vi "conversor-hex-car.vi"(10 "String":string) -> (2 "String 2":string)   [LabVIEW 2019]
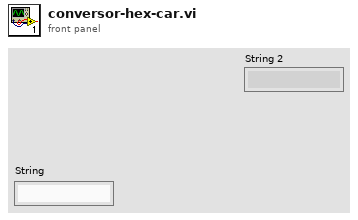
[diagram p1: front panel]
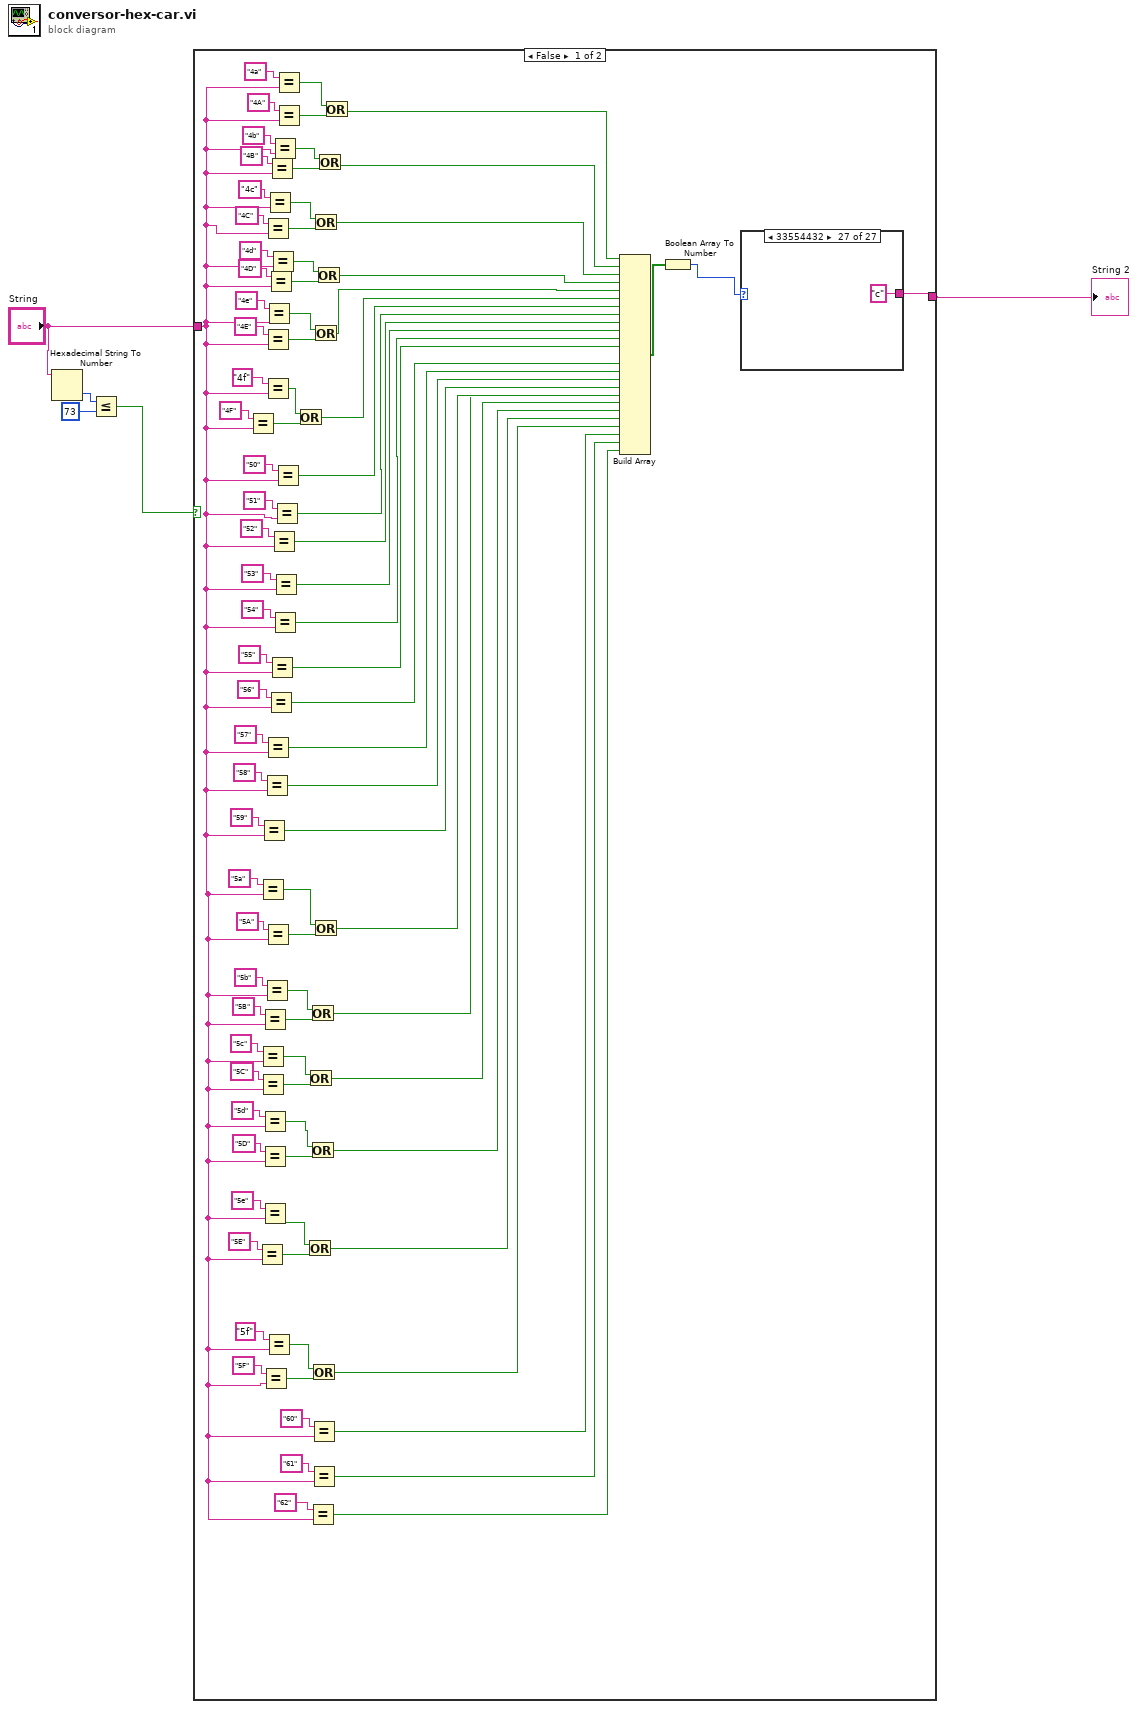
[diagram p0: block diagram]
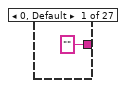
[diagram p2: hidden frame]
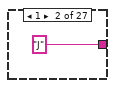
[diagram p3: hidden frame]
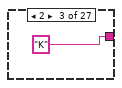
[diagram p4: hidden frame]
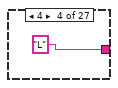
[diagram p5: hidden frame]
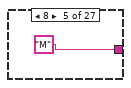
[diagram p6: hidden frame]
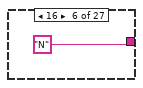
[diagram p7: hidden frame]
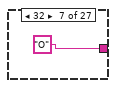
[diagram p8: hidden frame]
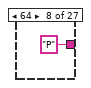
[diagram p9: hidden frame]
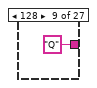
[diagram p10: hidden frame]
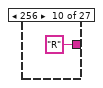
[diagram p11: hidden frame]
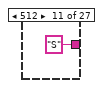
[diagram p12: hidden frame]
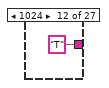
[diagram p13: hidden frame]
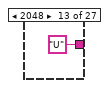
[diagram p14: hidden frame]
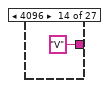
[diagram p15: hidden frame]
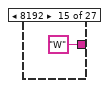
[diagram p16: hidden frame]
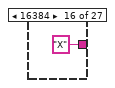
[diagram p17: hidden frame]
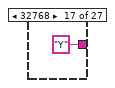
[diagram p18: hidden frame]
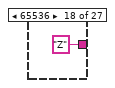
[diagram p19: hidden frame]
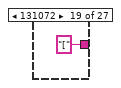
[diagram p20: hidden frame]
diagram:
  n1 = Hexadecimal String To Number(string="String") -> (number=w5:u32)  [unwired: 2 in, 1 out]
  n2 = Less Or Equal?(x=w5, y=u32 73) -> (x <= y?=w3:bool)
  n3 = case shown="False" w3 {
    tunnel: [w56 w188] -> w1
    tunnel: "String" -> [w8 w125]
    frame False {
      n4 = Equal?(x="4F", y=w8) -> (x = y?=w34:bool)
      n5 = Equal?(x="5E", y=w8) -> (x = y?=w14:bool)
      n6 = Equal?(x="5a", y=w8) -> (x = y?=w28:bool)
      n7 = Equal?(x="5c", y=w8) -> (x = y?=w20:bool)
      n8 = Equal?(x="5C", y=w8) -> (x = y?=w22:bool)
      n9 = Equal?(x="59", y=w8) -> (x = y?=w69:bool)
      n10 = Equal?(x="5B", y=w8) -> (x = y?=w26:bool)
      n11 = Equal?(x="5d", y=w8) -> (x = y?=w16:bool)
      n12 = Equal?(x="5D", y=w8) -> (x = y?=w18:bool)
      n13 = Equal?(x="5e", y=w8) -> (x = y?=w12:bool)
      n14 = Equal?(x="5F", y=w8) -> (x = y?=w10:bool)
      n15 = Equal?(x="58", y=w8) -> (x = y?=w70:bool)
      n16 = Equal?(x="5b", y=w8) -> (x = y?=w24:bool)
      n17 = Equal?(x="4C", y=w8) -> (x = y?=w46:bool)
      n18 = Equal?(x="4E", y=w8) -> (x = y?=w38:bool)
      n19 = Equal?(x="4f", y=w8) -> (x = y?=w32:bool)
      n20 = Equal?(x="57", y=w8) -> (x = y?=w71:bool)
      n21 = Equal?(x="5A", y=w8) -> (x = y?=w30:bool)
      n22 = Equal?(x="4e", y=w8) -> (x = y?=w36:bool)
      n23 = Equal?(x="5f", y=w8) -> (x = y?=w7:bool)
      n24 = Equal?(x="4c", y=w8) -> (x = y?=w44:bool)
      n25 = Equal?(x="4D", y=w8) -> (x = y?=w42:bool)
      n26 = Equal?(x="56", y=w8) -> (x = y?=w72:bool)
      n27 = Equal?(x="4B", y=w8) -> (x = y?=w50:bool)
      n28 = Equal?(x="55", y=w8) -> (x = y?=w77:bool)
      n29 = Equal?(x="4d", y=w8) -> (x = y?=w40:bool)
      n30 = Equal?(x="52", y=w8) -> (x = y?=w80:bool)
      n31 = Equal?(x="4b", y=w8) -> (x = y?=w48:bool)
      n32 = Equal?(x="54", y=w8) -> (x = y?=w78:bool)
      n33 = Equal?(x="53", y=w8) -> (x = y?=w79:bool)
      n34 = Equal?(x="51", y=w8) -> (x = y?=w81:bool)
      n35 = Equal?(x="50", y=w8) -> (x = y?=w82:bool)
      n36 = Equal?(x="4a", y=w8) -> (x = y?=w52:bool)
      n37 = Equal?(x="4A", y=w8) -> (x = y?=w54:bool)
      n38 = Or(x=w32, y=w34) -> (x .or. y?=w31:bool)
      n39 = Or(x=w12, y=w14) -> (x .or. y?=w11:bool)
      n40 = Or(x=w20, y=w22) -> (x .or. y?=w19:bool)
      n41 = Or(x=w24, y=w26) -> (x .or. y?=w23:bool)
      n42 = Or(x=w16, y=w18) -> (x .or. y?=w15:bool)
      n43 = Equal?(x="62", y=w8) -> (x = y?=w57:bool)
      n44 = Or(x=w7, y=w10) -> (x .or. y?=w6:bool)
      n45 = Equal?(x="60", y=w8) -> (x = y?=w59:bool)
      n46 = Equal?(x="61", y=w8) -> (x = y?=w58:bool)
      n47 = Or(x=w44, y=w46) -> (x .or. y?=w43:bool)
      n48 = Or(x=w36, y=w38) -> (x .or. y?=w35:bool)
      n49 = Or(x=w28, y=w30) -> (x .or. y?=w27:bool)
      n50 = Or(x=w40, y=w42) -> (x .or. y?=w39:bool)
      n51 = Or(x=w48, y=w50) -> (x .or. y?=w47:bool)
      n52 = Or(x=w52, y=w54) -> (x .or. y?=w51:bool)
      n53 = Build Array(w51, w47, w43, w39, w35, w31, w82, w81, w80, w79, w78, w77, w72, w71, w70, w69, w27, w23, w19, w15, w11, w6, w59, w58, w57) -> (w92:bool[])
      n54 = Boolean Array To Number(Boolean array=w92) -> (number=w55:u32)
      n55 = case shown="33554432" w55 {
        tunnel: ["" "J" "K" "L" "M" "N" "O" "P" "Q" "R" "S" "T" "U" "V" "W" "X" "Y" "Z" "[" "\\" "]" "^" "_" "`" "a" "b" "c"] -> w56
        frame 0, Default {
        }
        frame 1 {
        }
        frame 2 {
        }
        frame 4 {
        }
        frame 8 {
        }
        frame 16 {
        }
        frame 32 {
        }
        frame 64 {
        }
        frame 128 {
        }
        frame 256 {
        }
        frame 512 {
        }
        frame 1024 {
        }
        frame 2048 {
        }
        frame 4096 {
        }
        frame 8192 {
        }
        frame 16384 {
        }
        frame 32768 {
        }
        frame 65536 {
        }
        frame 131072 {
        }
        frame 262144 {
        }
        frame 524288 {
        }
        frame 1048576 {
        }
        frame 2097152 {
        }
        frame 4194304 {
        }
        frame 8388608 {
        }
        frame 16777216 {
        }
        frame 33554432 {
        }
      }
    }
    frame True {
      n56 = Equal?(x="3E", y=w125) -> (x = y?=w131:bool)
      n57 = Equal?(x="3D", y=w125) -> (x = y?=w135:bool)
      n58 = Equal?(x="3e", y=w125) -> (x = y?=w129:bool)
      n59 = Equal?(x="3C", y=w125) -> (x = y?=w139:bool)
      n60 = Equal?(x="3d", y=w125) -> (x = y?=w133:bool)
      n61 = Equal?(x="3B", y=w125) -> (x = y?=w143:bool)
      n62 = Equal?(x="3c", y=w125) -> (x = y?=w137:bool)
      n63 = Equal?(x="3b", y=w125) -> (x = y?=w141:bool)
      n64 = Equal?(x="3A", y=w125) -> (x = y?=w147:bool)
      n65 = Equal?(x="38", y=w125) -> (x = y?=w173:bool)
      n66 = Equal?(x="3a", y=w125) -> (x = y?=w145:bool)
      n67 = Equal?(x="35", y=w125) -> (x = y?=w182:bool)
      n68 = Equal?(x="39", y=w125) -> (x = y?=w172:bool)
      n69 = Equal?(x="37", y=w125) -> (x = y?=w174:bool)
      n70 = Equal?(x="32", y=w125) -> (x = y?=w191:bool)
      n71 = Equal?(x="36", y=w125) -> (x = y?=w175:bool)
      n72 = Equal?(x="34", y=w125) -> (x = y?=w183:bool)
      n73 = Equal?(x="33", y=w125) -> (x = y?=w184:bool)
      n74 = Equal?(x="31", y=w125) -> (x = y?=w192:bool)
      n75 = Equal?(x="30", y=w125) -> (x = y?=w193:bool)
      n76 = Equal?(x="3F", y=w125) -> (x = y?=w127:bool)
      n77 = Equal?(x="3f", y=w125) -> (x = y?=w124:bool)
      n78 = Equal?(x="48", y=w125) -> (x = y?=w149:bool)
      n79 = Equal?(x="49", y=w125) -> (x = y?=w148:bool)
      n80 = Equal?(x="47", y=w125) -> (x = y?=w150:bool)
      n81 = Equal?(x="46", y=w125) -> (x = y?=w151:bool)
      n82 = Equal?(x="45", y=w125) -> (x = y?=w152:bool)
      n83 = Equal?(x="44", y=w125) -> (x = y?=w153:bool)
      n84 = Equal?(x="41", y=w125) -> (x = y?=w156:bool)
      n85 = Equal?(x="43", y=w125) -> (x = y?=w154:bool)
      n86 = Equal?(x="42", y=w125) -> (x = y?=w155:bool)
      n87 = Equal?(x="40", y=w125) -> (x = y?=w157:bool)
      n88 = Or(x=w129, y=w131) -> (x .or. y?=w128:bool)
      n89 = Or(x=w133, y=w135) -> (x .or. y?=w132:bool)
      n90 = Or(x=w137, y=w139) -> (x .or. y?=w136:bool)
      n91 = Or(x=w141, y=w143) -> (x .or. y?=w140:bool)
      n92 = Or(x=w145, y=w147) -> (x .or. y?=w144:bool)
      n93 = Or(x=w124, y=w127) -> (x .or. y?=w123:bool)
      n94 = Build Array(w193, w192, w191, w184, w183, w182, w175, w174, w173, w172, w144, w140, w136, w132, w128, w123, w157, w156, w155, w154, w153, w152, w151, w150, w149, w148) -> (w190:bool[])
      n95 = Boolean Array To Number(Boolean array=w190) -> (number=w189:u32)
      n96 = case shown="0, Default" w189 {
        tunnel: ["" "0" "1" "2" "3" "4" "5" "6" "7" "8" "9" ":" ";" "<" "=" ">" "?" "@" "A" "B" "C" "D" "E" "F" "G" "H" "I"] -> w188
        frame 0, Default {
        }
        frame 1 {
        }
        frame 2 {
        }
        frame 4 {
        }
        frame 8 {
        }
        frame 16 {
        }
        frame 32 {
        }
        frame 64 {
        }
        frame 128 {
        }
        frame 256 {
        }
        frame 512 {
        }
        frame 1024 {
        }
        frame 2048 {
        }
        frame 4096 {
        }
        frame 8192 {
        }
        frame 16384 {
        }
        frame 32768 {
        }
        frame 65536 {
        }
        frame 131072 {
        }
        frame 262144 {
        }
        frame 524288 {
        }
        frame 1048576 {
        }
        frame 2097152 {
        }
        frame 4194304 {
        }
        frame 8388608 {
        }
        frame 16777216 {
        }
        frame 33554432 {
        }
      }
    }
  }
  "String 2" <- w1
